vi "Read VISA.vi"(8 "error in (no error)":errorcluster, 11 "MFC in":refnum<class "Sensor.lvclass">) -> (0 "error out":errorcluster, 2 "VISA 1":refnum<visa-resource-name>, 3 "MFC out":refnum<class "Sensor.lvclass">)   [LabVIEW 2013, in "Sensor.lvib.lvlib" / "Sensor.lvclass"]
uses:
  Sensor.lvclass
  Sensor.lvclass/Sensor.ctl
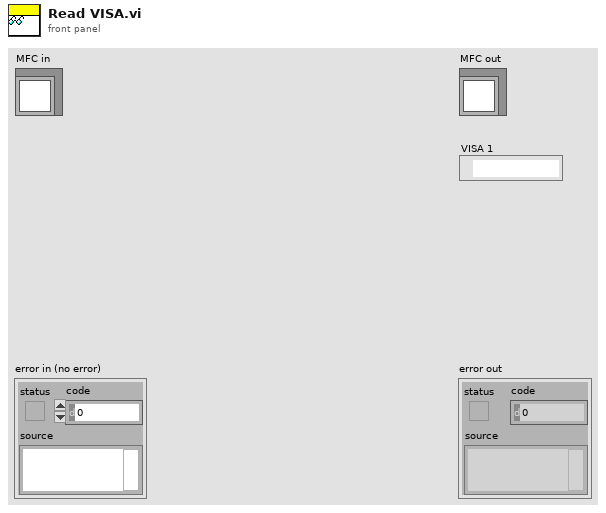
[diagram p1: front panel]
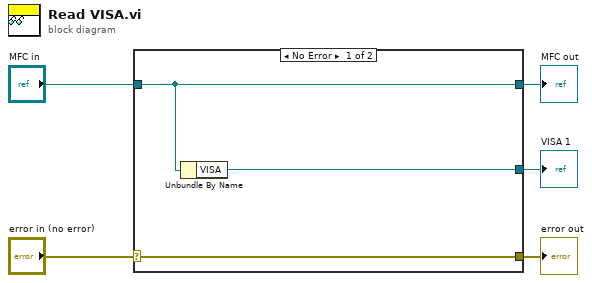
[diagram p0: block diagram]
diagram:
  n1 = case shown="No Error" "error in (no error)" {
    selector: "error in (no error)" -> [w8 w9]
    tunnel: [w8 w9] -> w4
    tunnel: [w7 w10] -> w2
    tunnel: "MFC in" -> [w7 w10]
    tunnel: [w6 _] -> w1
    frame No Error {
      n2 = Unbundle By Name(w7) -> ("VISA"=w6:refnum<visa-resource-name>)
    }
    frame Error {
    }
  }
  "error out" <- w4
  "MFC out" <- w2
  "VISA 1" <- w1
